vi "Parse Event Selector For Broadcast.vi"(7 "Config":refnum<class "TAF Proj Config.lvclass">, 11 "Event Selector":string) -> (3 "Broadcast Events":string[](array[string]))   [LabVIEW 2021, in "TAF Proj Document Type.lvlib" / "Project Parser.lvlib"]
uses:
  <vilib>/Wovalab/AntiDoc/Document Type/Add-ons/LabVIEW TAF Project/Project Parser/Project Parser.lvlib
  <vilib>/Wovalab/AntiDoc/Document Type/Add-ons/LabVIEW TAF Project/TAF Proj Config/TAF Proj Config.lvclass
  <vilib>/regexp/Match Regular Expression.xnode
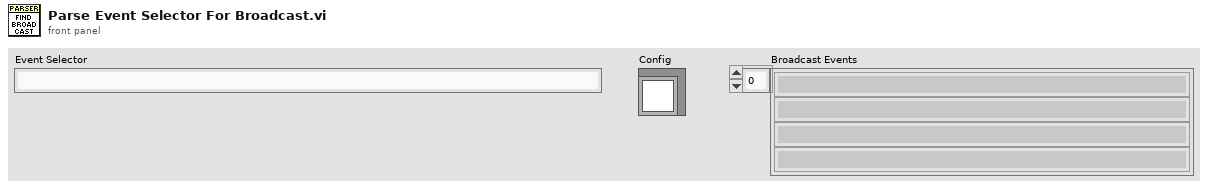
[diagram p1: front panel]
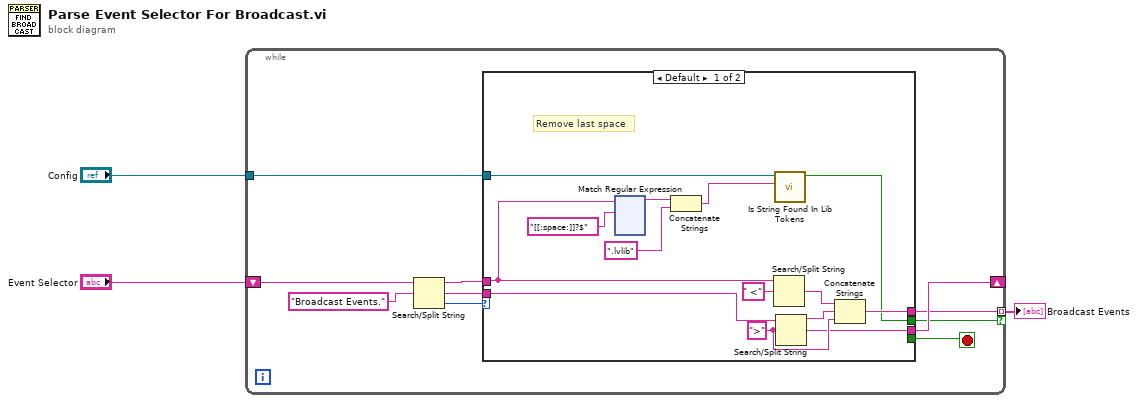
[diagram p0: block diagram]
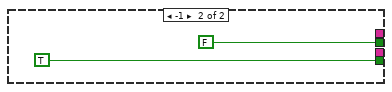
[diagram p2: hidden frame]
diagram:
  n1 = while {
    shift-right: [w7] -> _
    shift-left: "Event Selector" -> [w12]
    tunnel: [w6] -> w2 mode=indexing if=w5
    tunnel: "Config" -> [w4]
    stop <- w10 stop-if-true
    n2 = Search/Split String(string=w12, search string/char (-)="Broadcast Events.") -> (substring before match=w9:string, match + rest of string=w8:string, offset of match=w11:i32)  [unwired: 1 in]
    n3 = case shown="Default" w11 {
      tunnel: [_ TRUE] -> w10
      tunnel: w9 -> [w18 _]
      tunnel: w8 -> [w26 _]
      tunnel: [w22 _] -> w7
      tunnel: [w21 _] -> w6
      tunnel: [w19 FALSE] -> w5
      tunnel: w4 -> [w20 _]
      frame Default {
        w23 = ">" ("search string/char (-)")
        # "Remove last space"
        n4 = xnode "Match Regular Expression"("input string"=w18, "regular expression"="[[:space:]]?$") -> ("before match"=w14:string)  [unwired: 4 in, 4 out]
        n5 = Concatenate Strings(w14, ".lvlib" ("string")) -> (w16:string)
        n6 = Search/Split String(string=w18, search string/char (-)=" <") -> (match + rest of string=w25:string)  [unwired: 1 in, 2 out]
        n7 = call <vilib>:"Is String Found In Lib Tokens.vi"("String"=w16, "Config"=w20) -> ("Not Found?"=w19:bool)  [unwired: 9 in]
        n8 = Search/Split String(string=w26, search string/char (-)=w23) -> (substring before match=w24:string, match + rest of string=w22:string)  [unwired: 1 in, 1 out]
        n9 = Concatenate Strings(w25, w24, w23) -> (w21:string)
      }
      frame -1 {
      }
    }
  }
  "Broadcast Events" <- w2
